vi "List-Items To ID and Name.vi"(9 "Separate Sign":string="-", 11 "List in":refnum<vi>) -> (0 "Name":string=".ACS Units Group 0", 2 "ID":i64, 3 "List Out":refnum<vi>)   [LabVIEW 2024]
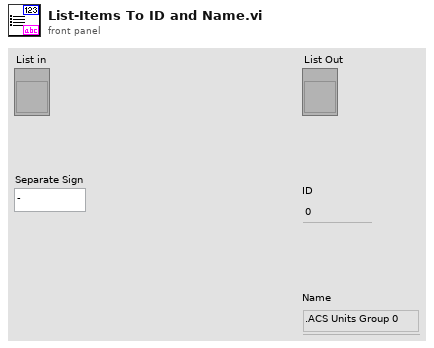
[diagram p1: front panel]
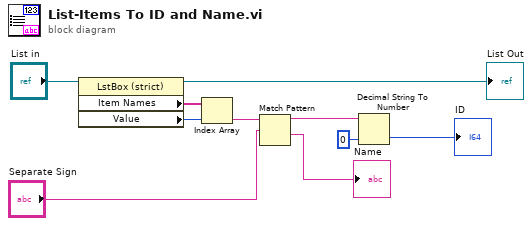
[diagram p0: block diagram]
diagram:
  n1 = property class="LstBox (strict)"(reference="List in") -> (reference out=→"List Out":refnum<vi>, "Item Names"=w10:string[], "Value"=w9:i32)  [unwired: 1 in, 1 out]
  n2 = Index Array(array=w10, index=w9) -> (element=w6:string)
  n3 = Match Pattern(string=w6, regular expression="Separate Sign") -> (before substring=w4:string, after substring=→"Name":string)  [unwired: 1 in, 2 out]
  n4 = Decimal String To Number(string=w4, default (0L)=i64 0 ("default (0 I32)")) -> (number=→"ID":i64)  [unwired: 1 in, 1 out]
